vi "CSMP-Unregister Status.vi"(0 "State":string, 1 "Args":string, 2 "Source/target":string, 5 "Error In":errorcluster caption="error in (no error)", 7 "CSMQ In":T1={"info"={"Module Name"="", "Requested Name"="", "Group Name"="", "Mode"=enum."Stand Alone", "Allowed Messages"=[]}, "Refs"={"WatchDogQ"=refnum, "CSMDataDVR"=refnum, "Queue"={"HPriorityQ"=refnum, "LowPriorityQ"=refnum}, "GroupDataDVR"=refnum, "TagMap"=refnum, "ExitEvent"=refnum, "NewStateEvent"=refnum, "StatusChangeEvent"=refnum}}, 8 "Module Name":string) -> (13 "CSMQ Out":T1={"info"={"Module Name"="", "Requested Name"="", "Group Name"="", "Mode"=enum."Stand Alone", "Allowed Messages"=[]}, "Refs"={"WatchDogQ"=refnum, "CSMDataDVR"=refnum, "Queue"={"HPriorityQ"=refnum, "LowPriorityQ"=refnum}, "GroupDataDVR"=refnum, "TagMap"=refnum, "ExitEvent"=refnum, "NewStateEvent"=refnum, "StatusChangeEvent"=refnum}}, 14 "State Out":string, 15 "Args Out":string, 16 "Source/target Out":string, 17 "Pre-State Out":string, 18 "Pre-Args Out":string, 19 "Error":errorcluster)   [LabVIEW 2017, in "Communicable State Machine.lvlib"]
doc: "### CSMP-Unregister Status.vi\n\n-- <b>Controls</b> --\n- <b>state</b>:\n- <b>args</b>:\n- <b>source/target</b>:\n- <b>Module Name</b>:\n\n-- <b>Indicators</b> --\n- <b>state out</b>:\n- <b>args out</b>:\n- <b>source/target out</b>:\n- <b>Pre-State out</b>:\n- <b>Pre-Args out</b>:\n- <b>error</b>:"
uses:
  Communicable State Machine.lvlib
  CSMQ/_CSMObj.ctl
  CSMQ/_CSMObj-Info.ctl
  Typedef/_CSM_MODE.ctl
  CSMQ/_CSMObj-Refs.ctl
  CSMQ/_CSMObj-Data.ctl
  Priority Queue/Priority Queue.ctl
  Typedef/_Cross CSM State Data.ctl
  Typedef/_CSM_MSG_TYPE.ctl
  Typedef/_Cross CSM State Response.ctl
  Typedef/_CSM_Response Source Message.ctl
  Priority Queue/def-Data(LowPRI-Q).ctl
  CSMQ/_CSMObj-ModeData.ctl
  Typedef/_CSM Status Change Event Data.ctl
  FGV-BroadcastRegistry/Operation-BroadcastRegistry.ctl
  AdvanceAPI/CSM - Make String Arguments Safe.vi
  AdvanceAPI/CSM - Keywords.vi
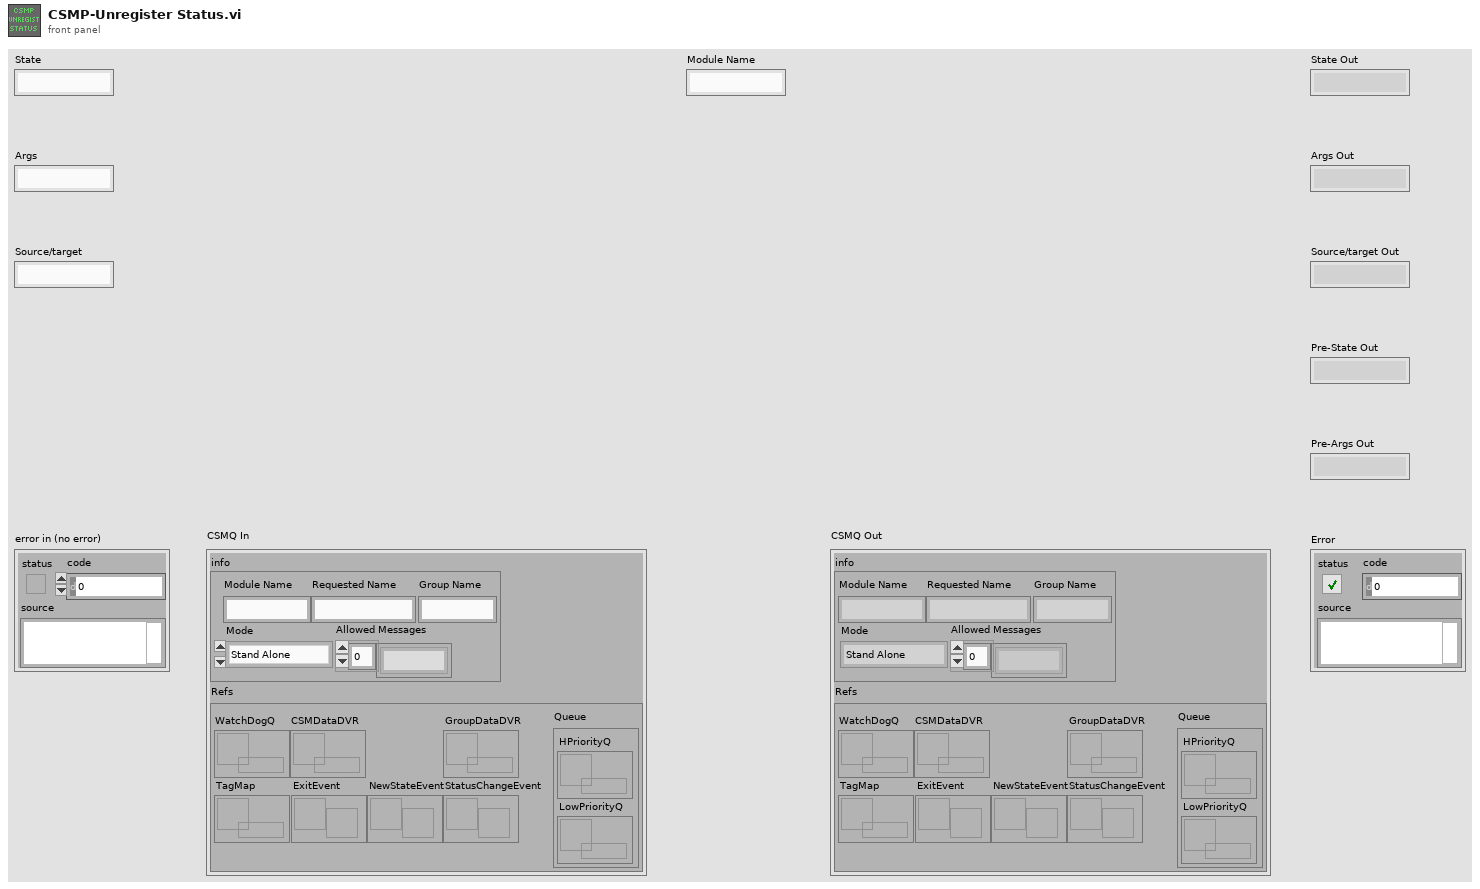
[diagram p1: front panel]
types:
  T1 = typedef "Communicable State Machine.lvlib/_CSMObj.ctl" = cluster{"info":T2, "Refs":T4}
  T2 = typedef "Communicable State Machine.lvlib/_CSMObj-Info.ctl" = cluster{"Module Name":string, "Requested Name":string, "Group Name":string, "Mode":T3, "Allowed Messages":string[]}
  T3 = typedef "Communicable State Machine.lvlib/_CSM_MODE.ctl" = enum16{"Not Exist", "Stand Alone", "CSM", "Worker", "Worker Agent", "Chain Node", "Chain"}
  T4 = typedef "Communicable State Machine.lvlib/_CSMObj-Refs.ctl" = cluster{"WatchDogQ":refnum<queue>, "CSMDataDVR":refnum<data-value>, "Queue":T5, "GroupDataDVR":refnum<data-value>, "TagMap":refnum<data-value>, "ExitEvent":refnum<user-event>, "NewStateEvent":refnum<user-event>, "StatusChangeEvent":refnum<user-event>}
  T5 = typedef "Communicable State Machine.lvlib/Priority Queue.ctl" = cluster{"HPriorityQ":refnum<queue>, "LowPriorityQ":refnum<queue>}
  T6 = typedef "Communicable State Machine.lvlib/Operation-BroadcastRegistry.ctl" = enum16{"Delete Source Module", "Delete Target Module", "Remove Module", "Register", "Unregister", "Check", "List Status", "List Entries", "List Status Of Source"}
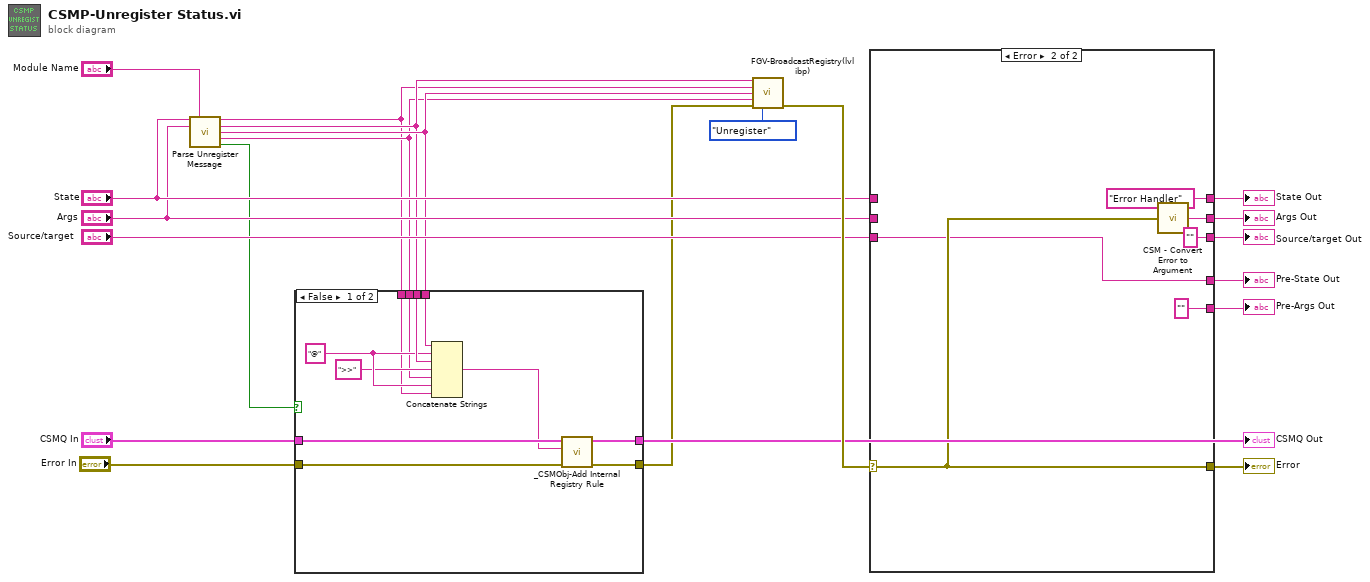
[diagram p0: block diagram]
diagram:
  n1 = call "Parse Unregister Message.vi"("State"="State", "Module Name"="Module Name", "Args"="Args") -> ("Target"=w3:string, "Source"=w5:string, "Status"=w6:string, "Api"=w4:string, "Target Specified?"=w2:bool)  [unwired: 8 in]
  n2 = case shown="False" w2 {
    tunnel: w6 -> [w32 _]
    tunnel: w5 -> [w31 _]
    tunnel: w4 -> [w28 _]
    tunnel: w3 -> [w27 _]
    tunnel: [w26 w34] -> w9
    tunnel: "CSMQ In" -> [w25 w34]
    tunnel: [w23 w33] -> w8
    tunnel: "Error In" -> [w22 w33]
    frame False {
      w30 = "@" ("string")
      n3 = Concatenate Strings(w32, w30, w31, ">>" ("string"), w28, w30, w27) -> (w24:string)
      n4 = call "_CSMObj-Add Internal Registry Rule.vi"("Error In"=w22, "Rule"=w24, "CSMQ In"=w25) -> ("error out"=w23:errorcluster, "CSMQ Out"=w26:T1)  [unwired: 7 in]
    }
    frame True {
    }
  }
  "CSMQ Out" <- w9
  n5 = call "FGV-BroadcastRegistry(lvlibp).vi"("Source"=w5, "Target"=w3, "Status"=w6, "API"=w4, "Error In"=w8, "Operation"=Operation-BroadcastRegistry."Unregister") -> ("error out"=w20:errorcluster)  [unwired: 8 in, 1 out]
  n6 = case shown="Error" w20 {
    selector: w20 -> [w35 w39]
    tunnel: [_ w37] -> w21
    tunnel: [w35 w39] -> w19
    tunnel: [_ "" ("Pre-State out")] -> w18
    tunnel: "State" -> [_ _]
    tunnel: [_ "Error Handler" ("state")] -> w17
    tunnel: "Args" -> [_ _]
    tunnel: [_ w38] -> w16
    tunnel: "Source/target" -> [_ w37]
    tunnel: [_ "" ("source/target")] -> w14
    frame No Error {
    }
    frame Error {
      n7 = call "CSM - Convert Error to Argument.vi"("Error"=w39) -> ("Argument"=w38:string)  [unwired: 4 in]
    }
  }
  "State Out" <- w17
  "Args Out" <- w16
  "Source/target Out" <- w14
  "Pre-State Out" <- w21
  "Pre-Args Out" <- w18
  "Error" <- w19
